vi "Query Trigger Event Overrun Status.vi"(8 "error in (no error)":errorcluster, 9 "Trigger Number (1)":i32=1, 10 "Trigger Type (2: Timer)":i32(ring)=2 items=["Digital IO", "Blender", "Timer", "TSP Link", "LAN"], 11 "VISA resource name":refnum<visa-resource-name>) -> (0 "error out":errorcluster, 2 "Event Overrun":bool, 3 "VISA resource name out":refnum<visa-resource-name>)   [LabVIEW 2015, in "Keithley 2600 Series.lvlib"]
doc: "Indicates whether or not an event was ignored because of the event detector state."
uses:
  Keithley 2600 Series.lvlib
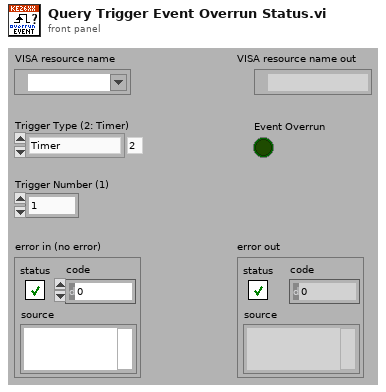
[diagram p1: front panel]
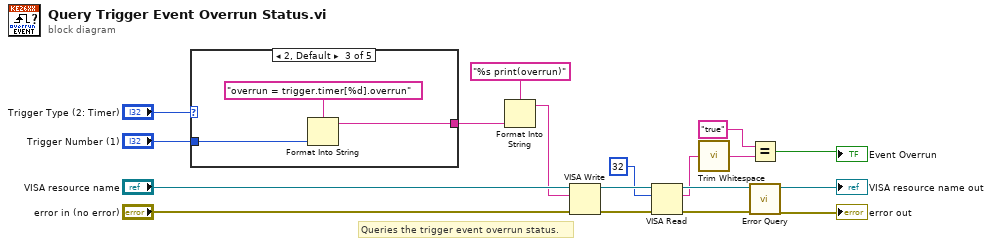
[diagram p0: block diagram]
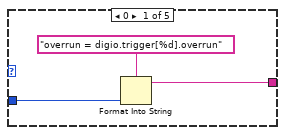
[diagram p2: hidden frame]
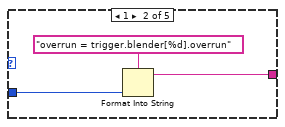
[diagram p3: hidden frame]
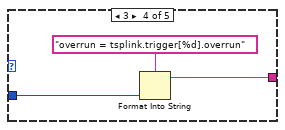
[diagram p4: hidden frame]
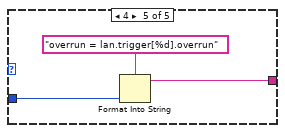
[diagram p5: hidden frame]
diagram:
  # "Queries the trigger event overrun status."
  n1 = case shown="2, Default" "Trigger Type (2: Timer)" {
    tunnel: "Trigger Number (1)" -> [w20 w23 w25 w28 w32]
    tunnel: [w19 w22 w26 w29 w31] -> w11
    frame 0 {
      n2 = Format Into String(format string="overrun = digio.trigger[%d].overrun", w20) -> (resulting string=w19:string)  [unwired: 2 in, 1 out]
    }
    frame 1 {
      n3 = Format Into String(format string="overrun = trigger.blender[%d].overrun", w23) -> (resulting string=w22:string)  [unwired: 2 in, 1 out]
    }
    frame 2, Default {
      n4 = Format Into String(format string="overrun = trigger.timer[%d].overrun", w25) -> (resulting string=w26:string)  [unwired: 2 in, 1 out]
    }
    frame 3 {
      n5 = Format Into String(format string="overrun = tsplink.trigger[%d].overrun", w28) -> (resulting string=w29:string)  [unwired: 2 in, 1 out]
    }
    frame 4 {
      n6 = Format Into String(format string="overrun = lan.trigger[%d].overrun", w32) -> (resulting string=w31:string)  [unwired: 2 in, 1 out]
    }
  }
  n7 = Format Into String(format string="%s print(overrun)", w11) -> (resulting string=w10:string)  [unwired: 2 in, 1 out]
  n8 = VISA Write(VISA resource name="VISA resource name", write buffer=w10, error in (no error)="error in (no error)") -> (VISA resource name out=w9:refnum<visa-resource-name>, error out=w8:errorcluster)  [unwired: 1 out]
  n9 = VISA Read(VISA resource name=w9, byte count=u32 32, error in (no error)=w8) -> (VISA resource name out=w7:refnum<visa-resource-name>, read buffer=w3:string, error out=w6:errorcluster)  [unwired: 1 out]
  n10 = call <vilib>:"Trim Whitespace.vi"("string"=w3) -> ("trimmed string"=w2:string)  [unwired: 1 in]
  n11 = Equal?(x="true", y=w2) -> (x = y?=→"Event Overrun":bool)
  n12 = call "Error Query.vi"("error in (no error)"=w6, "VISA resource name"=w7) -> ("error out"=→"error out":errorcluster, "VISA resource name out"=→"VISA resource name out":refnum<visa-resource-name>)  [unwired: 6 in, 2 out]
